vi "Convert freq-shift.vi"(9 "ADC Sample Rate [Hz]":dbl=1600000000.0 format="%#_13p", 10 "Frequency Shift (Hz)":dbl[](array[numeric]) format="%#_6p") -> (1 "Decimation Factor":dbl[](array[numeric]), 2 "ddc.freq.shift":fxp<+/-,48,0>[](array[numeric]) format="%.48g")   [LabVIEW 2015, in "7976R_v1.lvclass"]
uses:
  <userlib>/SE-APP-Receiver/NI5772/7976R_v1/7976R_v1.lvclass
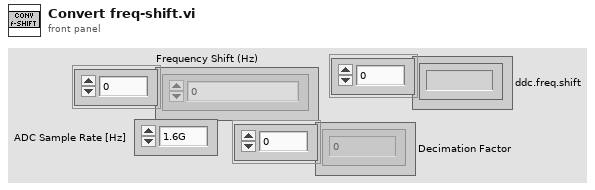
[diagram p1: front panel]
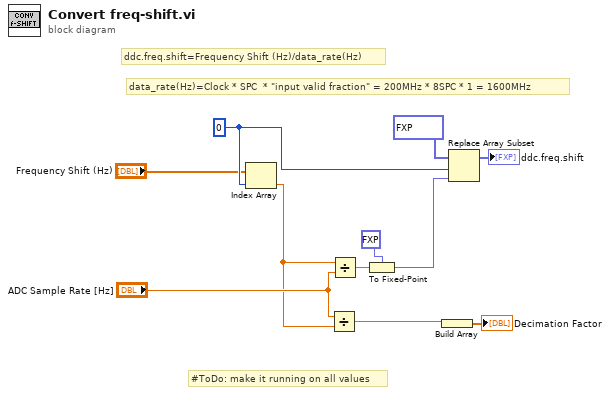
[diagram p0: block diagram]
diagram:
  w10 = 0 ("index")
  # "#ToDo: make it running on all values"
  # "data_rate(Hz)=Clock * SPC  * \"input valid fraction\" = 200MHz * 8SPC * 1 = 1600MHz"
  # "ddc.freq.shift=Frequency Shift (Hz)/data_rate(Hz)"
  n1 = Index Array(array="Frequency Shift (Hz)", index=w10) -> (element=w3:dbl)
  n2 = Divide(x="ADC Sample Rate [Hz]", y=w3) -> (x/y=w2:dbl)
  n3 = Divide(x=w3, y="ADC Sample Rate [Hz]") -> (x/y=w9:dbl)
  n4 = To Fixed-Point(fixed-point type=fxp<+/-,48,0> 0.0 ("ddc.freq.shift"), number=w9) -> (fixed-point=w11:fxp<+/-,48,0>)
  n5 = Build Array(w2) -> (→"Decimation Factor":dbl[])
  n6 = Replace Array Subset(array=fxp<+/-,48,0>[] [0.0, 0.0, 0.0, 0.0, 0.0, 0.0, 0.0, 0.0, 0.0, 0.0, 0.0, 0.0, 0.0, 0.0, 0.0, 0.0] ("ddc.freq.shift"), new element=w11, index=w10) -> (→"ddc.freq.shift":fxp<+/-,48,0>[])
